vi "UpdateControlsFromMCListbox.vi"(8 "error in (no error)":errorcluster, 10 "MulticolumnListbox in":refnum<vi>, 11 "Controls in":T1[](array[typedef])) -> (0 "error out":errorcluster)   [LabVIEW 2020, in "ContextHelpEditor.lvlib"]
uses:
  ContextHelpEditor.lvlib
  ControlRef--cluster.ctl
  <vilib>/picture/picture.llb/imagedata.ctl
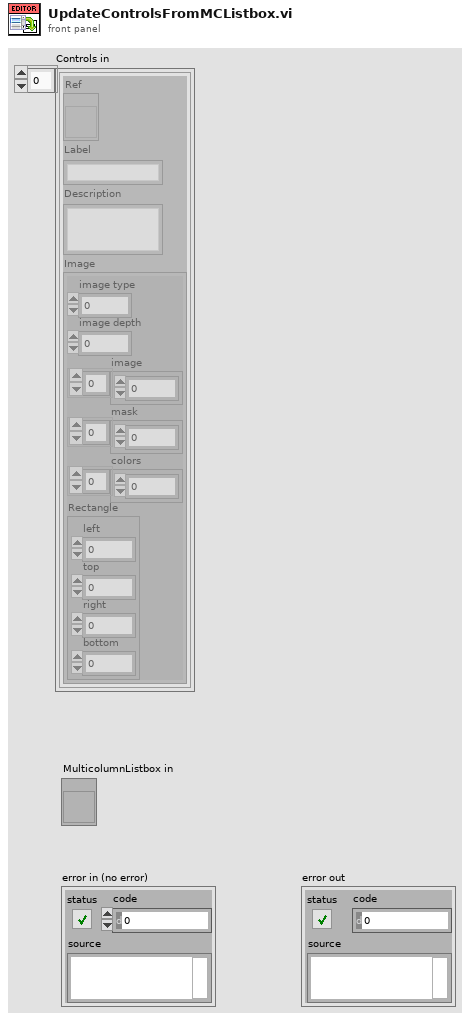
[diagram p1: front panel]
types:
  T1 = typedef "ContextHelpEditor.lvlib/ControlRef--cluster.ctl" = cluster{"Ref":refnum<vi>, "Label":string, "Description":string, "Image":T2}
  T2 = typedef "imagedata.ctl" = cluster{"image type":i32, "image depth":i32, "image":u8[], "mask":u8[], "colors":u32[], "Rectangle":cluster{"left":i16, "top":i16, "right":i16, "bottom":i16}}
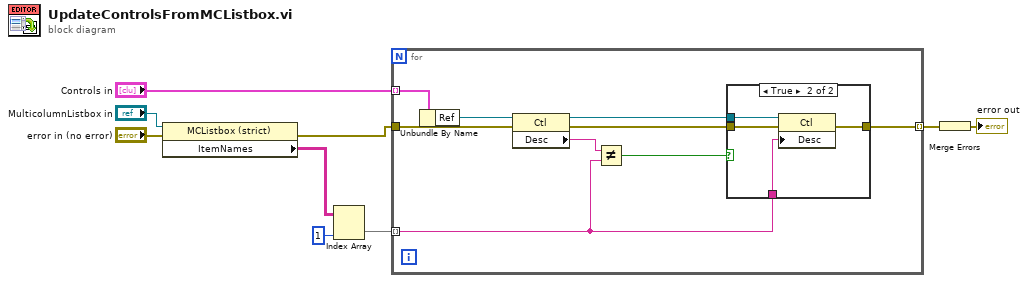
[diagram p0: block diagram]
diagram:
  n1 = property class="MCListbox (strict)"(reference="MulticolumnListbox in", error in="error in (no error)") -> (error out=w8:errorcluster, "ItemNames"=w5:string[][])  [unwired: 1 out]
  n2 = Index Array(array=w5, index (col)=1 ("disabled index (col)")) -> (element=w7:string[])  [unwired: 1 in]
  n3 = for {
    tunnel: "Controls in" -> [w18] mode=indexing
    tunnel: w8 -> [w14]
    tunnel: [w17] -> w3 mode=indexing
    tunnel: w7 -> [w11] mode=indexing
    n4 = Unbundle By Name(w18) -> ("Ref"=w16:refnum<vi>)
    n5 = property class="Ctl"(reference=w16, error in=w14) -> (reference out=w15:refnum<vi>, error out=w13:errorcluster, "Desc"=w12:string)
    n6 = Not Equal?(x=w12, y=w11) -> (x != y?=w10:bool)
    n7 = case shown="True" w10 {
      tunnel: [w19 w23] -> w17
      tunnel: w15 -> [_ w22]
      tunnel: w13 -> [w19 w21]
      tunnel: w11 -> [_ w20]
      frame False {
      }
      frame True {
        n8 = property class="Ctl"(reference=w22, error in=w21, "Desc"=w20) -> (error out=w23:errorcluster)  [unwired: 1 out]
      }
    }
  }
  n9 = Merge Errors(w3) -> (→"error out":errorcluster)
